vi "NN_Predict(In3D_Out3D)(CuLab).vi"(6 "Dataset":T1={"Dataset_Size"=0, "Dims_In"={"C"=0, "H"=0, "W"=0}, "Labels"=[], "File Paths"=[], "Outputs Ref."=refnum, "Inputs Ref."=variant(refnum<data-value> refnum), "Dims_Out"={"C"=0, "H"=0, "W"=0}}, 8 "error in (no error)":errorcluster, 11 "NN in":T4={"Name"="", "No of Layers"=0, "mBatch"=0, "Layers"=[], "Dimty"=enum."In1D_Out1D", "Dims_In"={"C"=0, "H"=0, "W"=0}, "Dims_Out"={"C"=0, "H"=0, "W"=0}, "Working_Dir"=path "", "Train?"=FALSE, "Train_Params"={"Optimizer"=enum."SGD", "Beta_1"=0.0, "Beta_2"=0.0, "Weight Decay(L1)"=0.0, "Weight Decay(L2)"=0.0, "Data_Sampling"=enum."Random"}, "LR_Update_Policy"={"Policy_Type"=enum."Manual", "LR0"=0.0, "k"=0.0, "WarmUp_Policy"=enum."Step", "WarmUp_Iter"=100, "WarmUp_Ratio"=10.0}, "Session Data"={"Epochs"=0.0, "Tot_Iter"=0, "LR"=0.0, "LR_iter"=0}, "Ground_truth"={"Y"=variant(refnum<data-value> refnum)}, "NNg_hdls"={"cudnn"=0, "cublas"=0, "stream"=0, "curand"=0}, "NN_Device"=enum."CPU", "GPU Id"=0, "Labels"=[], "Receptive Field"=[], "Loss_Type"=enum."MSE", "Loss_Cfg_Prms"=variant, "NNG_WS"={"NNG_WS_Mem"=refnum, "Max_WS_Size"=0}} {"LR_Update_Policy"."WarmUp_Ratio" min=1; "LR_Update_Policy"."WarmUp_Iter" min=1; "LR_Update_Policy"."LR0" format="%.7f"}) -> (0 "error out":errorcluster, 2 "Predictions Tensor":refnum<class "T4D_SGL.lvclass">, 3 "NN out":T4={"Name"="", "No of Layers"=0, "mBatch"=0, "Layers"=[], "Dimty"=enum."In1D_Out1D", "Dims_In"={"C"=0, "H"=0, "W"=0}, "Dims_Out"={"C"=0, "H"=0, "W"=0}, "Working_Dir"=path "", "Train?"=FALSE, "Train_Params"={"Optimizer"=enum."SGD", "Beta_1"=0.0, "Beta_2"=0.0, "Weight Decay(L1)"=0.0, "Weight Decay(L2)"=0.0, "Data_Sampling"=enum."Random"}, "LR_Update_Policy"={"Policy_Type"=enum."Manual", "LR0"=0.0, "k"=0.0, "WarmUp_Policy"=enum."Step", "WarmUp_Iter"=100, "WarmUp_Ratio"=10.0}, "Session Data"={"Epochs"=0.0, "Tot_Iter"=0, "LR"=0.0, "LR_iter"=0}, "Ground_truth"={"Y"=variant(refnum<data-value> refnum)}, "NNg_hdls"={"cudnn"=0, "cublas"=0, "stream"=0, "curand"=0}, "NN_Device"=enum."CPU", "GPU Id"=0, "Labels"=[], "Receptive Field"=[], "Loss_Type"=enum."MSE", "Loss_Cfg_Prms"=variant, "NNG_WS"={"NNG_WS_Mem"=refnum, "Max_WS_Size"=0}} {"LR_Update_Policy"."WarmUp_Ratio" min=1; "LR_Update_Policy"."WarmUp_Iter" min=1; "LR_Update_Policy"."LR0" format="%.7f"})   [LabVIEW 2020]
doc: "Runs forward propagation over whole dataset of type In3D_Out3D and returns prediction for a pretrained network.\n\n<b>NN in</b> - Network instance input.\n<b>Dataset</b> - A dataset of type In3D_Out3D for which predictions should be generated.\n<b>Predictions</b> - Contains feature maps of the last layer (predictions).\n<b>Predictions</b> - Returns predictions (network outputs) for applied dataset.\n<b>NN out</b> - Network instance output."
uses:
  <vilib>/Ngene/Deep Learning Toolkit/Toolkit/NN_Network/Controls/NN.ctl
  <vilib>/Ngene/Deep Learning Toolkit/Toolkit/NN_Layers/Controls/NN_Layer_ref.ctl
  <vilib>/Ngene/Deep Learning Toolkit/Toolkit/NN_Layers/Controls/NN_Layer.ctl
  <vilib>/Ngene/Deep Learning Toolkit/Toolkit/NN_Layers/Controls/NN_Layer_Type.ctl
  <vilib>/Ngene/Deep Learning Toolkit/Toolkit/NN_Data/API/NN_Dims(C,H,W).ctl
  <vilib>/Ngene/Deep Learning Toolkit/Toolkit/NN_Layers/Controls/NN_Layer_Metrics.ctl
  <vilib>/Ngene/Deep Learning Toolkit/Toolkit/NN_Network/Controls/NN_Device.ctl
  <vilib>/Ngene/Deep Learning Toolkit/Toolkit/NNg/cuda/Controls/nng_cuda_handles.ctl
  <vilib>/Ngene/Deep Learning Toolkit/Toolkit/NN_Layers/Controls/NN_Layer_Dimty.ctl
  <vilib>/Ngene/Deep Learning Toolkit/Toolkit/NN_Layers/Controls/NN_Layer_RF_State.ctl
  <vilib>/Ngene/Deep Learning Toolkit/Toolkit/NN_Data/API/NN_Dims(V,H).ctl
  <vilib>/Ngene/Deep Learning Toolkit/Toolkit/NN_Network/Controls/NN_In_Out_Dim-ty.ctl
  <vilib>/Ngene/Deep Learning Toolkit/Toolkit/NN_Train/Controls/NN_Train_Params.ctl
  <vilib>/Ngene/Deep Learning Toolkit/Toolkit/NN_Train/Controls/NN_Train_Optimizer.ctl
  <vilib>/Ngene/Deep Learning Toolkit/Toolkit/NN_Train/Controls/NN_Train_Data_Sampling.ctl
  <vilib>/Ngene/Deep Learning Toolkit/Toolkit/NN_Train/Controls/NN_LR_Policy_Cfg.ctl
  <vilib>/Ngene/Deep Learning Toolkit/Toolkit/NN_Train/Controls/NN_LR_Policy_Type.ctl
  <vilib>/Ngene/Deep Learning Toolkit/Toolkit/NN_Train/Controls/NN_Train_Session_Data.ctl
  <vilib>/Ngene/Deep Learning Toolkit/Toolkit/NN_Data/Controls/NN_Ground_truth.ctl
  <vilib>/Ngene/Deep Learning Toolkit/Toolkit/NN_Train/Controls/NN_Loss_Type.ctl
  <vilib>/Ngene/Deep Learning Toolkit/Toolkit/NNg/Network/WS/Controls/NNG_WS.ctl
  <vilib>/Ngene/Deep Learning Toolkit/Toolkit/NNg/Network/WS/Controls/NNg_WS_Mem_DVR.ctl
  <vilib>/Ngene/Deep Learning Toolkit/Toolkit/NNg/cuda/Controls/cuda_Mem_desc.ctl
  <vilib>/Ngene/Deep Learning Toolkit/Toolkit/NN_Data/API/DataSet/DataSet_Types/NN_DataSet(In3D_Out3D).ctl
  <vilib>/Ngene/Deep Learning Toolkit/Toolkit/NN_Data/Controls/DataRef_Types/4D/NN_Data_ref(4D_SGL).ctl
  <vilib>/Ngene/CuLab - GPU Accelerated Toolkit/Toolkit/Low_Level/Tensor_Classes/T_Children/T4D/T4D_Children/T4D_SGL/T4D_SGL.lvclass
  C:/Program Files/National Instruments/LabVIEW 2020/vi.lib/Ngene/CuLab - GPU Accelerated Toolkit/Toolkit/Low_Level/Tensor_Classes/T_Children/T4D/T4D.lvclass
  C:/Program Files/National Instruments/LabVIEW 2020/vi.lib/Ngene/CuLab - GPU Accelerated Toolkit/Toolkit/Low_Level/Tensor_Classes/Tensor.lvclass
  <vilib>/Ngene/CuLab - GPU Accelerated Toolkit/Toolkit/Low_Level/Tensor_Classes/T_Children/T4D/Controls/T4D_Dims.ctl
  <vilib>/Ngene/CuLab - GPU Accelerated Toolkit/Toolkit/Low_Level/Tensor_Classes/T_Children/T4D/Controls/T4D_Indices.ctl
  <vilib>/Ngene/CuLab - GPU Accelerated Toolkit/Toolkit/API/Array/Array Size/CU_Array_Size_T4D.vi
  <vilib>/Ngene/CuLab - GPU Accelerated Toolkit/Toolkit/API/Array/Initialize Array/T4D/CU_Initialize Array_T4D_SGL.vi
  <vilib>/Ngene/Deep Learning Toolkit/Toolkit/Deep_Learning_Toolkit_by_Ngene.lvlib
  <vilib>/Ngene/CuLab - GPU Accelerated Toolkit/Toolkit/CuLab.lvlib
  <vilib>/Ngene/CuLab - GPU Accelerated Toolkit/Toolkit/Low_Level/Tensor_Classes/Tensor.lvclass
  C:/Program Files/National Instruments/LabVIEW 2020/vi.lib/Ngene/CuLab - GPU Accelerated Toolkit/Toolkit/Low_Level/Tensor_Classes/T_Children/T4D/T4D_Children/T4D_SGL/T4D_SGL.lvclass
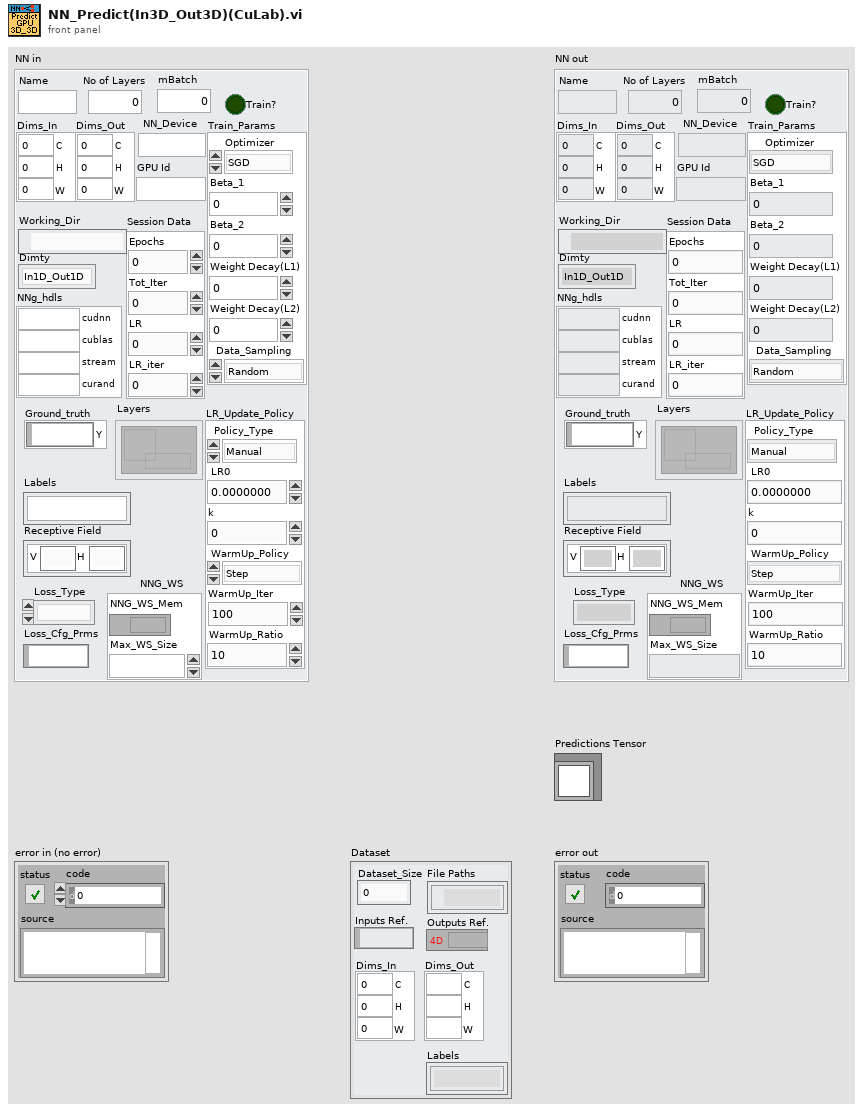
[diagram p1: front panel]
types:
  T1 = typedef "Deep_Learning_Toolkit_by_Ngene.lvlib/NN_DataSet(In3D_Out3D).ctl" = cluster{"Dataset_Size":i32, "Dims_In":T2, "Labels":string[], "File Paths":path[], "Outputs Ref.":T3, "Inputs Ref.":variant, "Dims_Out":T2}
  T2 = typedef "Deep_Learning_Toolkit_by_Ngene.lvlib/NN_Dims(C,H,W).ctl" = cluster{"C":i32, "H":i32, "W":i32}
  T3 = typedef "Deep_Learning_Toolkit_by_Ngene.lvlib/NN_Data_ref(4D_SGL).ctl" = refnum<data-value>
  T4 = typedef "Deep_Learning_Toolkit_by_Ngene.lvlib/NN.ctl" = cluster{"Name":string, "No of Layers":i32, "mBatch":i32, "Layers":T5[], "Dimty":T6, "Dims_In":T2, "Dims_Out":T2, "Working_Dir":path, "Train?":bool, "Train_Params":T7, "LR_Update_Policy":T10, "Session Data":T12, "Ground_truth":T13, "NNg_hdls":T14, "NN_Device":T15, "GPU Id":i32, "Labels":string[], "Receptive Field":T16[], "Loss_Type":T17, "Loss_Cfg_Prms":variant, "NNG_WS":T18}
  T5 = typedef "Deep_Learning_Toolkit_by_Ngene.lvlib/NN_Layer_ref.ctl" = refnum<data-value>
  T6 = typedef "Deep_Learning_Toolkit_by_Ngene.lvlib/NN_In_Out_Dim-ty.ctl" = enum8{"In1D_Out1D", "In3D_Out1D", "In3D_Out3D", "In3D_OutBBox"}
  T7 = typedef "Deep_Learning_Toolkit_by_Ngene.lvlib/NN_Train_Params.ctl" = cluster{"Optimizer":T8, "Beta_1":sgl, "Beta_2":sgl, "Weight Decay(L1)":sgl, "Weight Decay(L2)":sgl, "Data_Sampling":T9}
  T8 = typedef "Deep_Learning_Toolkit_by_Ngene.lvlib/NN_Train_Optimizer.ctl" = enum16{"SGD", "Adam", "Adagrad", "Adadelta", "RMSProp", "Nesterov"}
  T9 = typedef "Deep_Learning_Toolkit_by_Ngene.lvlib/NN_Train_Data_Sampling.ctl" = enum16{"Random", "Sequential"}
  T10 = typedef "Deep_Learning_Toolkit_by_Ngene.lvlib/NN_LR_Policy_Cfg.ctl" = cluster{"Policy_Type":T11, "LR0":dbl, "k":sgl, "WarmUp_Policy":enum16{"Step", "Ramp"}, "WarmUp_Iter":i32, "WarmUp_Ratio":sgl}
  T11 = typedef "Deep_Learning_Toolkit_by_Ngene.lvlib/NN_LR_Policy_Type.ctl" = enum16{"Manual", "Step", "Exp", "1/t"}
  T12 = typedef "Deep_Learning_Toolkit_by_Ngene.lvlib/NN_Train_Session_Data.ctl" = cluster{"Epochs":sgl, "Tot_Iter":i32, "LR":sgl, "LR_iter":i32}
  T13 = typedef "Deep_Learning_Toolkit_by_Ngene.lvlib/NN_Ground_truth.ctl" = cluster{"Y":variant}
  T14 = typedef "Deep_Learning_Toolkit_by_Ngene.lvlib/nng_cuda_handles.ctl" = cluster{"cudnn":u64, "cublas":u64, "stream":u64, "curand":u64}
  T15 = typedef "Deep_Learning_Toolkit_by_Ngene.lvlib/NN_Device.ctl" = enum16{"CPU", "GPU"}
  T16 = typedef "Deep_Learning_Toolkit_by_Ngene.lvlib/NN_Dims(V,H).ctl" = cluster{"V":i32, "H":i32}
  T17 = typedef "Deep_Learning_Toolkit_by_Ngene.lvlib/NN_Loss_Type.ctl" = enum16{"None", "MSE", "CrossEntropy", "YOLO_v2", "YOLO_v4"}
  T18 = typedef "Deep_Learning_Toolkit_by_Ngene.lvlib/NNG_WS.ctl" = cluster{"NNG_WS_Mem":T19, "Max_WS_Size":i64}
  T19 = typedef "Deep_Learning_Toolkit_by_Ngene.lvlib/NNg_WS_Mem_DVR.ctl" = refnum<data-value>
  T20 = typedef "CuLab.lvlib/T4D_Dims.ctl" = cluster{"N":i32, "C ":i32, "H":i32, "W":i32}
  T21 = typedef "CuLab.lvlib/T4D_Indices.ctl" = cluster{"n":i32, "k ":i32, "i":i32, "j":i32}
  T22 = typedef "Deep_Learning_Toolkit_by_Ngene.lvlib/NN_Layer.ctl" = cluster{"Name":string, "Layer_Data":variant, "Layer_Type":T23, "Dims_In":T2, "Layers_In":variant, "Dims_Out":T2, "Layers_Out":variant, "Metrics":T24, "GPU_Data":variant, "mBatch":i32, "NN_Device":T15, "NNg_hdls":T14, "Train?":bool, "Dimty":T25, "RecptField":T26}
  T23 = typedef "Deep_Learning_Toolkit_by_Ngene.lvlib/NN_Layer_Type.ctl" = enum16{"Input1D", "Input3D", "Conv1D", "Conv2D", "Conv2D_Adv", "MaxPool", "AvgPool", "UpSample", "DropOut3D", "ShortCut", "Concat", "SoftMax3D", "FC", "DropOut", "Softmax", "Flatten", "YOLO_v2", "YOLO_v4", "Activation", "BatchNormalization", "Unsupported"}
  T24 = typedef "Deep_Learning_Toolkit_by_Ngene.lvlib/NN_Layer_Metrics.ctl" = cluster{"Data":dbl, "Params":dbl, "Ops":dbl}
  T25 = typedef "Deep_Learning_Toolkit_by_Ngene.lvlib/NN_Layer_Dimty.ctl" = enum16{"1D", "3D"}
  T26 = typedef "Deep_Learning_Toolkit_by_Ngene.lvlib/NN_Layer_RF_State.ctl" = cluster{"Dims":T16, "J":T16}
  T27 = typedef "CuLab.lvlib/cudart_DataType.ctl" = enum16{"I8", "U8", "I16", "U16", "I32", "U32", "I64", "U64", "SGL", "DBL", "CSG", "CDB"}
  T28 = typedef "CuLab.lvlib/cudart_Mem_desc.ctl" = cluster{"Ref*":u64, "Size(B)":u64}
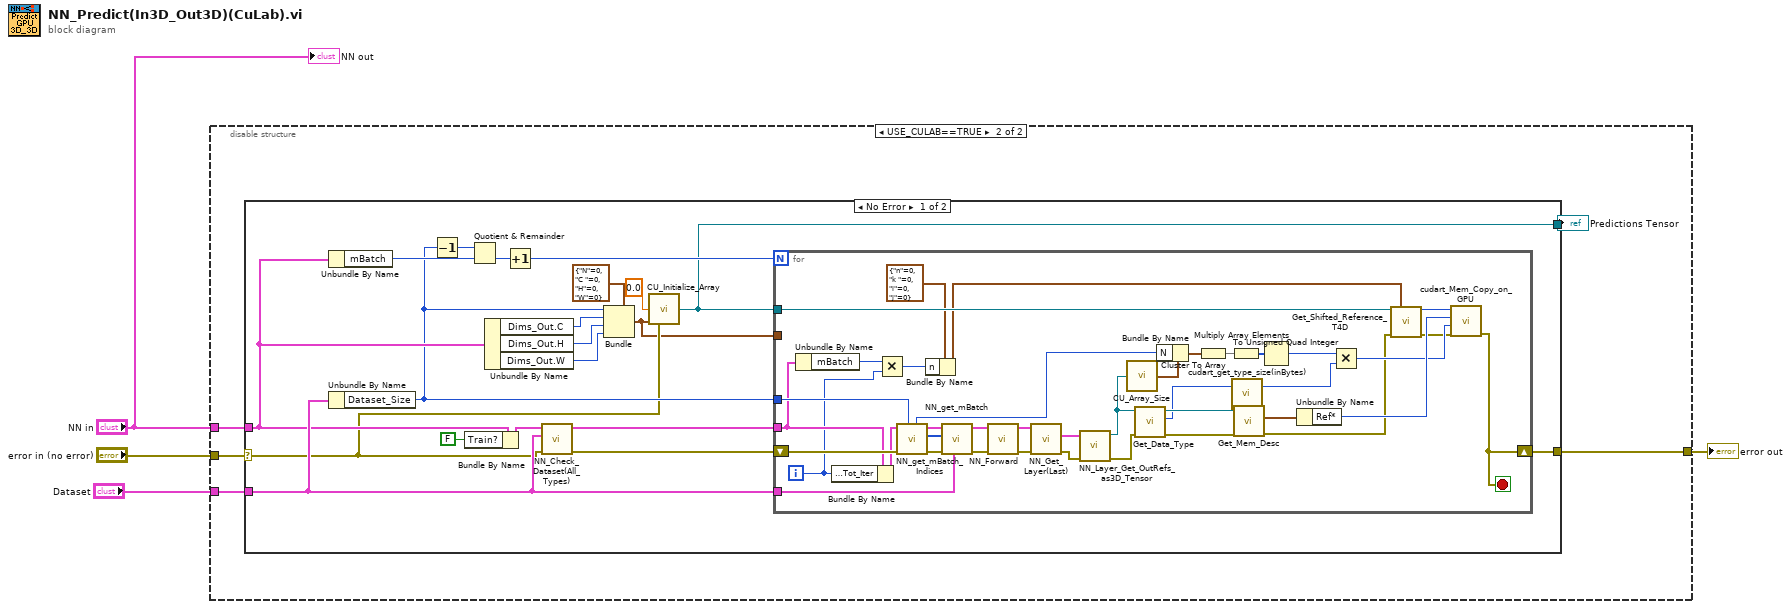
[diagram p0: block diagram]
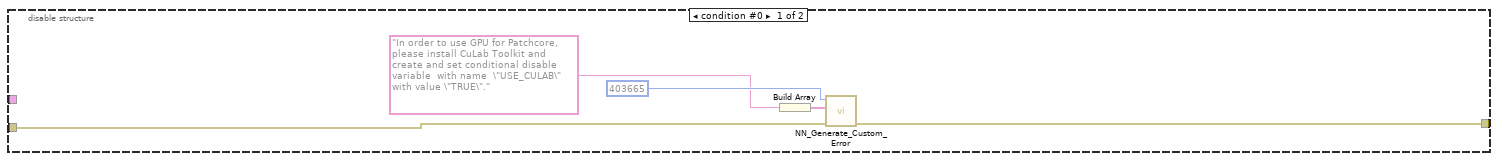
[diagram p2: hidden frame]
diagram:
  n1 = disable-structure shown="USE_CULAB==TRUE" {
    disable-tunnel: "Dataset" -> [_ w14]
    disable-tunnel: "NN in" -> [_ w13]
    disable-tunnel: "error in (no error)" -> [w6 w12]
    disable-tunnel: [w5 w10] -> w1
    frame condition #0 {
      n2 = Build Array("In order to use GPU for Patchcore, please install CuLab Toolkit and create and set conditional disable variable  with name  \"USE_CULAB\" with value \"TRUE\"." ("Message")) -> (w8:string[])
      n3 = call <vilib>:"NN_Generate_Custom_Error.vi"("error in (no error)"=w6, "Message"=w8, "Error_code"=403665) -> ("error out"=w5:errorcluster)  [unwired: 8 in]
    }
    frame condition #1 (active) {
      n4 = case shown="No Error" w12 {
        selector: w12 -> [w18 w74]
        tunnel: w14 -> [w25 _]
        tunnel: w13 -> [w23 _]
        tunnel: [w34 w74] -> w10
        tunnel: [w15 _] -> w11
        frame No Error {
          n5 = Unbundle By Name(w23) -> ("mBatch"=w28:i32)
          n6 = Unbundle By Name(w25) -> ("Dataset_Size"=w22:i32)
          n7 = Decrement(x=w22) -> (x-1=w31:i32)
          n8 = Bundle By Name(cluster=w23, "Train?"=FALSE) -> (w33:T4)
          n9 = Quotient & Remainder(x=w31, y=w28) -> (floor(x/y)=w30:i32)  [unwired: 1 out]
          n10 = Unbundle By Name(w23) -> ("Dims_Out.C"=w21:i32, "Dims_Out.H"=w20:i32, "Dims_Out.W"=w19:i32)
          n11 = Increment(x=w30) -> (x+1=w29:i32)
          n12 = call <vilib>:"NN_Check_Dataset(All_Types).vi"("error in (no error)"=w18, "Train DataSet"=w25, "NN in"=w33) -> ("error out"=w26:errorcluster, "NN out"=w27:T4)  [unwired: 5 in, 2 out]
          n13 = Bundle(cluster=T20 {"N"=0, "C "=0, "H"=0, "W"=0} ("dimension sizes"), "N"=w22, "C"=w21, "H"=w20, "W"=w19) -> (w17:T20)
          n14 = call-poly <vilib>:"CU_Initialize_Array.vi"("element"=sgl 0.0, "dimension sizes"=w17, "error in (no error)"=w18) -> ("initialized Tensor"=w15:refnum<class "T4D_SGL.lvclass">)  [unwired: 11 in, 1 out]
          n15 = for {
            N: w29 -> [_]
            shift-right: [w39] -> w34
            shift-left: w26 -> [w68]
            tunnel: w25 -> [w36]
            tunnel: w27 -> [w46]
            tunnel: w22 -> [w65]
            tunnel: w15 -> [w62]
            tunnel: w17 -> [_]
            i -> [w43]
            stop <- w39 stop-if-true
            n16 = Unbundle By Name(w46) -> ("mBatch"=w44:i32)
            n17 = Bundle By Name(cluster=w46, "Session Data.Tot_Iter"=w43) -> (w66:T4)
            n18 = Multiply(x=w44, y=w43) -> (x*y=w40:i32)
            n19 = call <vilib>:"NN_get_mBatch_Indices.vi"("Dataset_Size"=w65, "error in (no error)"=w68, "NN in"=w66) -> ("error out"=w67:errorcluster, "Indices"=w64:i32[], "NN Out"=w69:T4, "Actual mBatch Size"=w45:i32)  [unwired: 5 in]
            n20 = Bundle By Name(cluster=T21 {"n"=0, "k "=0, "i"=0, "j"=0} ("indices"), "n"=w40) -> (w41:T21)
            n21 = call <vilib>:"NN_get_mBatch.vi"("DataSet"=w36, "error in (no error)"=w67, "Indices"=w64, "NN in"=w69) -> ("error out"=w71:errorcluster, "NN Out"=w72:T4)  [unwired: 5 in, 1 out]
            n22 = call <vilib>:"NN_Forward.vi"("error in (no error)"=w71, "NN in"=w72) -> ("error out"=w70:errorcluster, "NN out"=w73:T4)  [unwired: 6 in, 2 out]
            n23 = call <vilib>:"NN_Get_Layer(Last).vi"("error in (no error)"=w70, "NN in"=w73) -> ("error out"=w61:errorcluster, "Last_Layer"=w63:T22)  [unwired: 6 in, 2 out]
            n24 = call "NN_Layer_Get_OutRefs_as3D_Tensor.vi"("error in (no error)"=w61, "Layer"=w63) -> ("error out"=w35:errorcluster, "Out"=w50:refnum<class "T4D_SGL.lvclass">)  [unwired: 7 in, 1 out]
            n25 = call-poly <vilib>:"CU_Array_Size.vi"("Tensor"=w50) -> ("T4D_Dims"=w49:T20)  [unwired: 14 in]
            n26 = call-dynamic "Get_Data_Type.vi"("error in (no error)"=w35, "T4D_SGL in"=w50) -> ("error out"=w38:errorcluster, "DataType"=w53:T27, "T4D_SGL out"=w54:refnum<class "T4D_SGL.lvclass">)  [unwired: 7 in]
            n27 = Bundle By Name(cluster=w49, "N"=w45) -> (w48:T20)
            n28 = Cluster To Array(cluster=w48) -> (array=w57:i32[])
            n29 = To Unsigned Quad Integer(1:w57) -> (0:w56:u64[])
            n30 = call <vilib>:"cudart_get_type_size(inBytes).vi"("DataType_t"=w53) -> ("Size in Bytes"=w52:u64)  [unwired: 2 in]
            n31 = call <vilib>:"Get_Mem_Desc.vi"("error in (no error)"=w38, "Tensor in"=w54) -> ("error out"=w37:errorcluster, "Mem_Desc"=w59:T28)  [unwired: 5 in, 3 out]
            n32 = Multiply Array Elements(1:w56) -> (0:w55:u64)
            n33 = Unbundle By Name(w59) -> ("Ref*"=w58:u64)
            n34 = Multiply(x=w55, y=w52) -> (x*y=w51:u64)
            n35 = call <vilib>:"Get_Shifted_Reference_T4D.vi"("Tensor"=w62, "indices"=w41, "error in (no error)"=w37) -> ("Ref* out"=w60:u64, "error out"=w47:errorcluster)  [unwired: 11 in]
            n36 = call <vilib>:"cudart_Mem_Copy_on_GPU.vi"("error in (no error)"=w47, "size"=w51, "src"=w58, "dest"=w60) -> ("error out"=w39:errorcluster)  [unwired: 6 in, 1 out]
          }
        }
        frame Error {
        }
      }
      "Predictions Tensor" <- w11
    }
  }
  "error out" <- w1
  "NN out" <- "NN in"
